vi "Sim Data.vi"(7 "QuWire in":refnum<class "QuWire.lvclass">) -> (4 "State Vector":cdb[](array[numeric]), 6 "Porababilities":dbl[](array[numeric]), 15 "Qubits n":i32)   [LabVIEW 2020]
uses:
  QuSim/QuWire/QuWire.lvclass
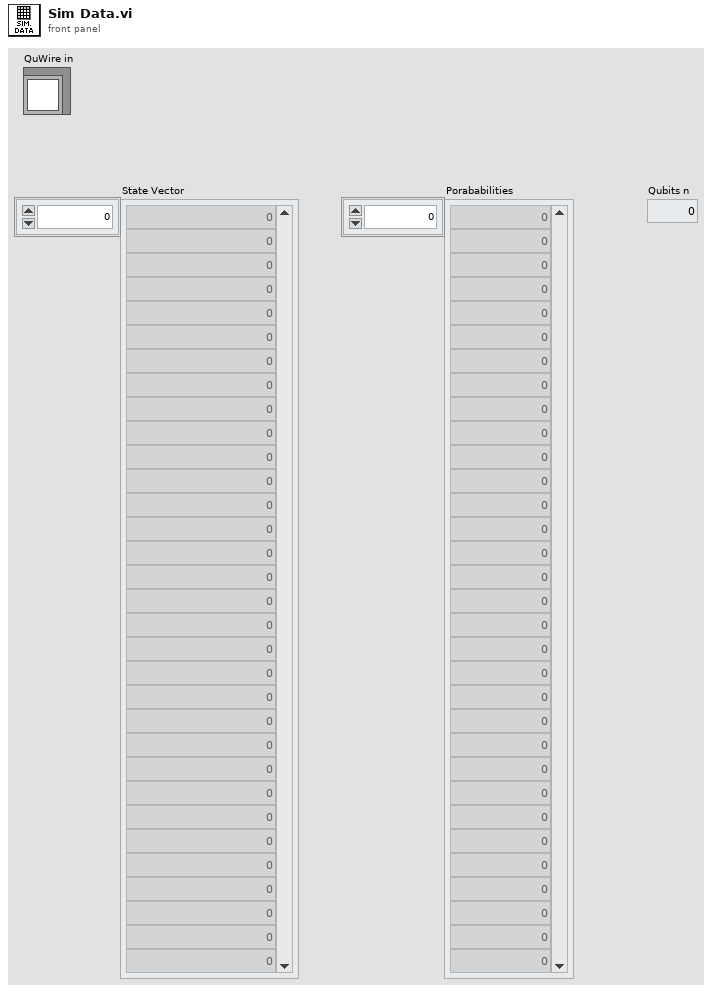
[diagram p1: front panel]
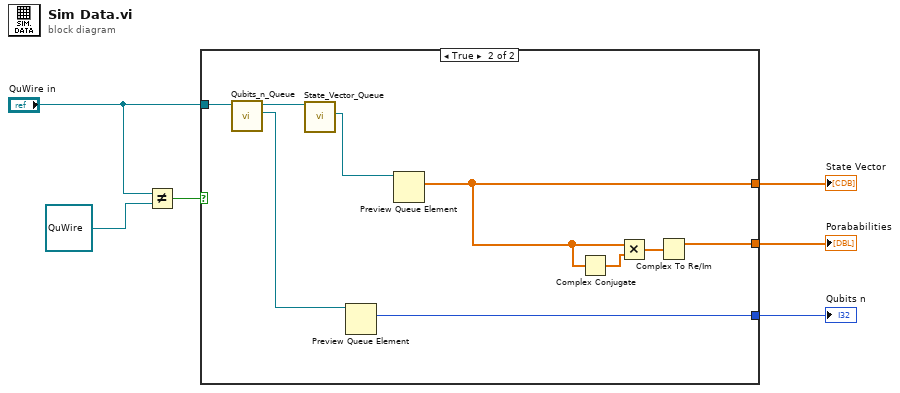
[diagram p0: block diagram]
diagram:
  n1 = Not Equal?(x="QuWire in", y=refnum<class "QuWire.lvclass"> refnum ("QuWire in")) -> (x != y?=w1:bool)
  n2 = case shown="True" w1 {
    tunnel: "QuWire in" -> [_ w14]
    tunnel: [_ w12] -> w6
    tunnel: [_ w8] -> w5
    tunnel: [_ w7] -> w4
    frame False {
    }
    frame True {
      n3 = call "Qubits_n_Queue.vi"("QuWire in"=w14) -> ("Qubit n"=w15:refnum<queue>, "QuWire out"=w13:refnum<class "QuWire.lvclass">)  [unwired: 8 in, 1 out]
      n4 = call "State_Vector_Queue.vi"("QuWire in"=w13) -> ("State Vector Queue"=w11:refnum<queue>)  [unwired: 8 in, 2 out]
      n5 = Preview Queue Element(queue=w15) -> (element=w12:i32)  [unwired: 2 in, 3 out]
      n6 = Preview Queue Element(queue=w11) -> (element=w8:cdb[])  [unwired: 2 in, 3 out]
      n7 = Complex Conjugate(1:w8) -> (0:w9:cdb[])
      n8 = Multiply(x=w8, y=w9) -> (x*y=w10:cdb[])
      n9 = Complex To Re/Im(x + iy=w10) -> (x=w7:dbl[])  [unwired: 1 out]
    }
  }
  "Qubits n" <- w6
  "State Vector" <- w5
  "Porababilities" <- w4
